vi "Report temperatures.vi"(8 "error in (no error)":errorcluster, 11 "VISA resource name":refnum<visa-resource-name>) -> (0 "error out":errorcluster, 2 "Temperatures":T1, 3 "VISA resource name out":refnum<visa-resource-name>)   [LabVIEW 2020, in "Marlin Instrument Driver.lvlib"]
doc: "Returns the current state of the configured X, Y, Z endstops. Takes into account any 'inverted endstop' settings, so one can confirm that the machine is interpreting the endstops correctly."
uses:
  <instrlib>/Marlin Instrument Driver/Marlin Instrument Driver.lvlib
  <instrlib>/Marlin Instrument Driver/Public/controls/temperatures.ctl
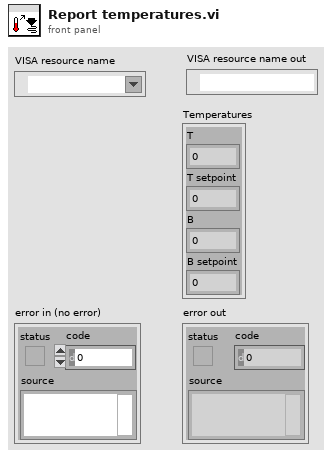
[diagram p1: front panel]
types:
  T1 = typedef "Marlin Instrument Driver.lvlib/temperatures.ctl" = cluster{"T":dbl, "T setpoint":dbl, "B":dbl, "B setpoint":dbl}
  T2 = cluster{"[0]":dbl, "[1]":dbl, "[2]":dbl, "[3]":dbl}
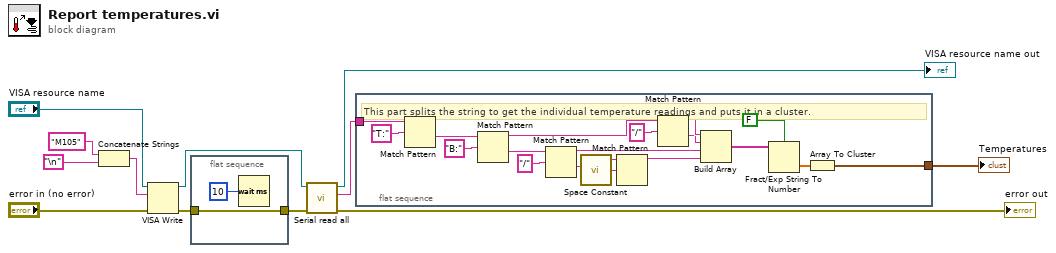
[diagram p0: block diagram]
diagram:
  n1 = Concatenate Strings("M105" ("command"), "\n") -> (w9:string)
  n2 = VISA Write(VISA resource name="VISA resource name", write buffer=w9, error in (no error)="error in (no error)") -> (VISA resource name out=w8:refnum<visa-resource-name>, error out=w2:errorcluster)  [unwired: 1 out]
  n3 = flat-sequence {
    tunnel: w2 -> [w13]
    tunnel: [w13] -> w1
    frame #0 {
      n4 = Wait (ms)(milliseconds to wait=u32 10) -> ()  [unwired: 1 out]
    }
  }
  n5 = call <instrlib>:"Serial read all.vi"("error in (no error)"=w1, "VISA Refnum in"=w8) -> ("error out"=→"error out":errorcluster, "read buffer"=w4:string, "VISA Refnum out"=→"VISA resource name out":refnum<visa-resource-name>)  [unwired: 6 in, 1 out]
  n6 = flat-sequence {
    tunnel: w4 -> [w32]
    tunnel: [w15] -> w3
    frame #0 {
      # "This part splits the string to get the individual temperature readings and puts it in a cluster."
      n7 = Match Pattern(string=w32, regular expression="T:") -> (after substring=w29:string)  [unwired: 1 in, 3 out]
      n8 = Match Pattern(string=w29, regular expression="B:") -> (before substring=w28:string, after substring=w25:string)  [unwired: 1 in, 2 out]
      n9 = Match Pattern(string=w25, regular expression="/") -> (before substring=w22:string, after substring=w21:string)  [unwired: 1 in, 2 out]
      n10 = call <vilib>:"Space Constant.vi"() -> ("String"=w20:string)
      n11 = Match Pattern(string=w21, regular expression=w20) -> (before substring=w19:string)  [unwired: 1 in, 3 out]
      n12 = Match Pattern(string=w28, regular expression="/") -> (before substring=w24:string, after substring=w23:string)  [unwired: 1 in, 2 out]
      n13 = Build Array(w24, w23, w22, w19) -> (w18:string[])
      n14 = Fract/Exp String To Number(use system decimal point (T)=FALSE, string=w18) -> (number=w16:dbl[])  [unwired: 2 in, 1 out]
      n15 = Array To Cluster(array=w16) -> (cluster=w15:T2)
    }
  }
  "Temperatures" <- w3
